vi "Day05-2.vi"() -> ()   [LabVIEW 2021]
panel:
  out "points with at least two lines overlap":i32
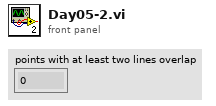
[diagram p1: front panel]
types:
  T1 = cluster{"[0]":i32, "[1]":i32, "[2]":i32, "[3]":i32, "[4]":i32, "[5]":i32, "[6]":i32, "[7]":i32, "[8]":i32}
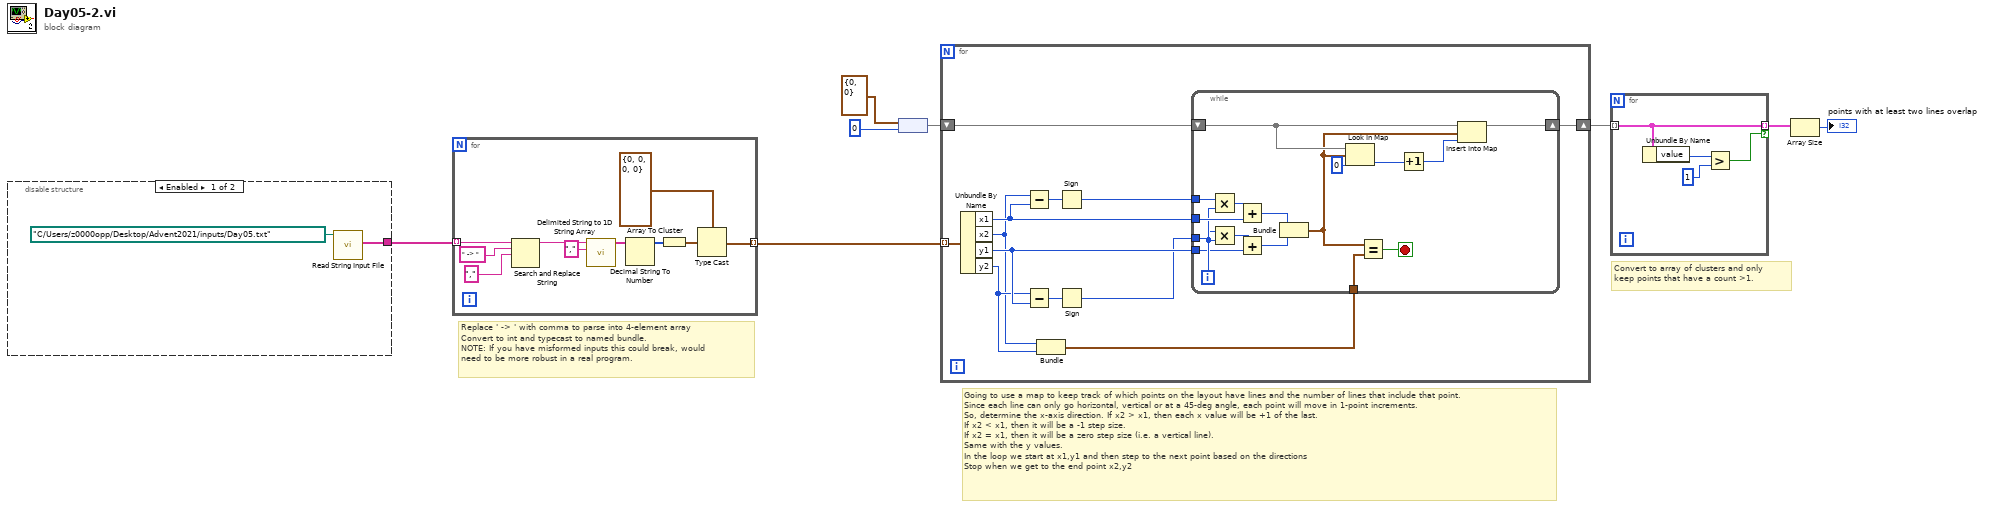
[diagram p0: block diagram]
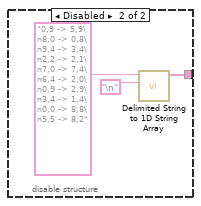
[diagram p2: hidden frame]
diagram:
  # "Convert to array of clusters and only\nkeep points that have a count >1."
  # "Going to use a map to keep track of which points on the layout have lines and the number of lines that include that point.\nSince each line can only go horizontal, vertical or at a 45-deg angle, each point will move in 1-point increments.\nSo, determine the x-axis direction. If x2 > x1, then each x value will be +1 of the last.\nIf x2 < x1, then it will be a -1 step size.\nIf x2 = x1, then it will be a zero step size (i.e. a vertical line).\nSame with the y values.\nIn the loop we start at x1,y1 and then step to the next point based on the directions\nStop when we get to the end point x2,y2"
  # "Replace ' -> ' with comma to parse into 4-element array\nConvert to int and typecast to named bundle.\nNOTE: If you have misformed inputs this could break, would\nneed to be more robust in a real program."
  n1 = disable-structure shown="Enabled" {
    disable-tunnel: [w9 w11] -> w8
    frame Enabled {
      n2 = call "Read String Input File.vi"("file path (dialog if empty)"=path "C:/Users/z0000opp/Desktop/Advent2021/inputs/Day05.txt") -> ("input values"=w9:string[])  [unwired: 10 in]
    }
    frame Disabled {
      n3 = call <vilib>:"Delimited String to 1D String Array.vi"("delimiter"="\n", "delimited string"="0,9 -> 5,9\n8,0 -> 0,8\n9,4 -> 3,4\n2,2 -> 2,1\n7,0 -> 7,4\n6,4 -> 2,0\n0,9 -> 2,9\n3,4 -> 1,4\n0,0 -> 8,8\n5,5 -> 8,2") -> ("string array"=w11:string[])  [unwired: 9 in]
    }
  }
  n4 = for {
    tunnel: w8 -> [w23] mode=indexing
    tunnel: [w14] -> w1 mode=indexing
    n5 = Search and Replace String(input string=w23, search string=" -> ", replace string=",") -> (result string=w20:string)  [unwired: 5 in, 3 out]
    n6 = call <vilib>:"Delimited String to 1D String Array.vi"("delimiter"=",", "delimited string"=w20) -> ("string array"=w18:string[])  [unwired: 9 in]
    n7 = Decimal String To Number(string=w18) -> (number=w17:i32[])  [unwired: 2 in, 1 out]
    n8 = Array To Cluster(array=w17) -> (cluster=w16:T1)
    n9 = Type Cast(type=cluster{"x1":i32, "y1":i32, "x2":i32, "y2":i32} {"x1"=0, "y1"=0, "x2"=0, "y2"=0}, x=w16) -> (*(type *) &x=w14:cluster{"x1":i32, "y1":i32, "x2":i32, "y2":i32})
  }
  n10 = node(cluster{"x":i32, "y":i32} {"x"=0, "y"=0}, 0) -> (w7:map{cluster{"x":i32, "y":i32}, i32})
  n11 = for {
    tunnel: w1 -> [w33] mode=indexing
    shift-right: [w34] -> w4
    shift-left: w7 -> [w35]
    n12 = Unbundle By Name(w33) -> ("x1"=w30:i32, "x2"=w25:i32, "y1"=w29:i32, "y2"=w26:i32)
    n13 = Subtract(x=w25, y=w30) -> (x-y=w32:i32)
    n14 = Subtract(x=w26, y=w29) -> (x-y=w31:i32)
    n15 = Bundle("x2"=w25, "y2"=w26) -> (w24:cluster{"x2":i32, "y2":i32})  [unwired: 1 in]
    n16 = Sign(1:w32) -> (0:w28:i32)
    n17 = Sign(1:w31) -> (0:w27:i32)
    n18 = while {
      shift-right: [w48] -> w34
      shift-left: w35 -> [w51]
      tunnel: w30 -> [w47]
      tunnel: w29 -> [w41]
      tunnel: w28 -> [w46]
      tunnel: w27 -> [w42]
      tunnel: w24 -> [w37]
      i -> [w43]
      stop <- w36 stop-if-true
      n19 = Multiply(x=w46, y=w43) -> (x*y=w45:i32)
      n20 = Multiply(x=w42, y=w43) -> (x*y=w44:i32)
      n21 = Add(x=w45, y=w47) -> (x+y=w40:i32)
      n22 = Add(x=w44, y=w41) -> (x+y=w39:i32)
      n23 = Bundle(w40, w39) -> (w38:cluster{i32, i32})  [unwired: 1 in]
      n24 = Look In Map(map=w51, key=w38, default value=0) -> (value=w50:i32)  [unwired: 1 out]
      n25 = Equal?(x=w38, y=w37) -> (x = y?=w36:bool)
      n26 = Increment(x=w50) -> (x+1=w49:i32)
      n27 = Insert Into Map(map in=w51, key=w38, value=w49) -> (map out=w48:map{cluster{"x":i32, "y":i32}, i32})  [unwired: 2 out]
    }
  }
  n28 = for {
    tunnel: [w56] -> w3 mode=indexing if=w53
    tunnel: w4 -> [w56] mode=indexing
    n29 = Unbundle By Name(w56) -> ("value"=w55:i32)
    n30 = Greater?(x=w55, y=1) -> (0:w53:bool)
  }
  n31 = Array Size(array=w3) -> (size(s)=→"points with at least two lines overlap":i32)
